vi "physics_lab.vi"() -> ()   [LabVIEW 2019]
panel:
  out "Display":dbl
  in  "stop":bool
  in  "phi":dbl
  in  "f":dbl
  in  "m":dbl
  in  "b":dbl
  in  "Ao":dbl(knob) scale=0.0..10.0
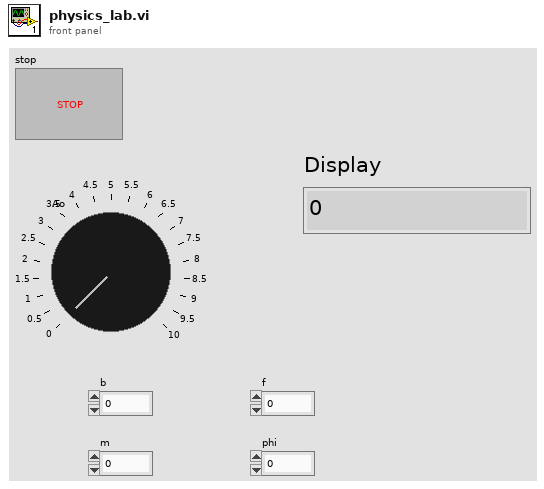
[diagram p1: front panel]
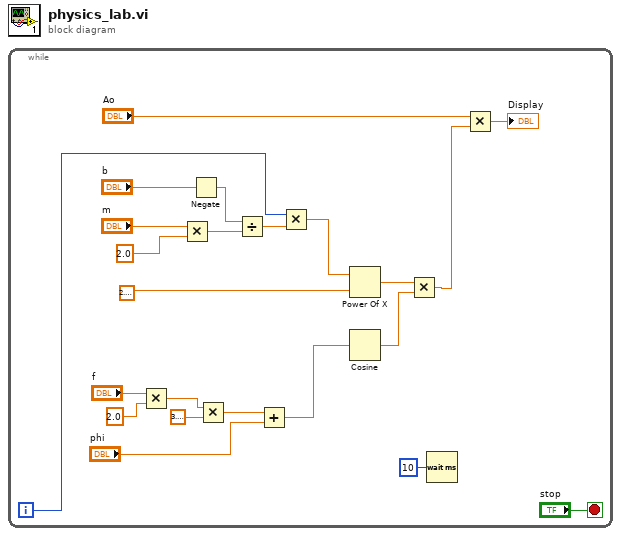
[diagram p0: block diagram]
diagram:
  n1 = while {
    i -> [w4]
    stop <- "stop" stop-if-true
    n2 = Multiply(x="f", y=2.0) -> (x*y=w11:dbl)
    n3 = Multiply(x="m", y=2.0) -> (x*y=w21:dbl)
    n4 = Negate(x="b") -> (-x=w19:dbl)
    n5 = Multiply(x=w11, y=3.141592653589793) -> (x*y=w8:dbl)
    n6 = Divide(x=w19, y=w21) -> (x/y=w16:dbl)
    n7 = Add(x=w8, y="phi") -> (x+y=w6:dbl)
    n8 = Multiply(x=w4, y=w16) -> (x*y=w15:dbl)
    n9 = Power Of X(1:2.718281828459045, 2:w15) -> (0:w14:dbl)
    n10 = Cosine(x=w6) -> (cos(x)=w13:dbl)
    n11 = Multiply(x=w14, y=w13) -> (x*y=w3:dbl)
    n12 = Wait (ms)(milliseconds to wait=u32 10) -> ()  [unwired: 1 out]
    n13 = Multiply(x="Ao", y=w3) -> (x*y=→"Display":dbl)
  }
